vi "Set PMD wrapper.vi"(6 "pDummyPMDInfoOut":cluster{"uiPwmDuty1":u8, "uiPwmDuty2":u8}, 7 "bAckEna":i32, 8 "error in (no error)":errorcluster caption="错误输入（无错误）", 9 "pDummyPMDInfoIn":cluster{"uiPwmDuty1":u8, "uiPwmDuty2":u8}, 10 "dwCanNodeId":u32, 11 "dwDevIndex":u32) -> (0 "error out":errorcluster caption="错误输出", 1 "pDummyPMDInfoIn out":cluster{"uiPwmDuty1":u8, "uiPwmDuty2":u8}, 3 "function return":u32, 4 "pDummyPMDInfoOut out":cluster{"uiPwmDuty1":u8, "uiPwmDuty2":u8})   [LabVIEW 2016, in "UISimCanFunc_wrapper.lvlib"]
doc: "_declspec (dllexport) DWORD SetPMD_wrapper(DWORD dwDevIndex, DWORD dwCanNodeId,\n P_DUMMY_PMD_INFO_OBJ pDummyPMDInfoIn, BOOL bAckEna, P_DUMMY_PMD_INFO_OBJ pDummyPMDInfoOut);"
uses:
  <userlib>/UISimCanFunc_wrapper/UISimCanFunc_wrapper.lvlib
  <userlib>/UISimCanFunc_wrapper/UISimCanFunc_wrapper.dll
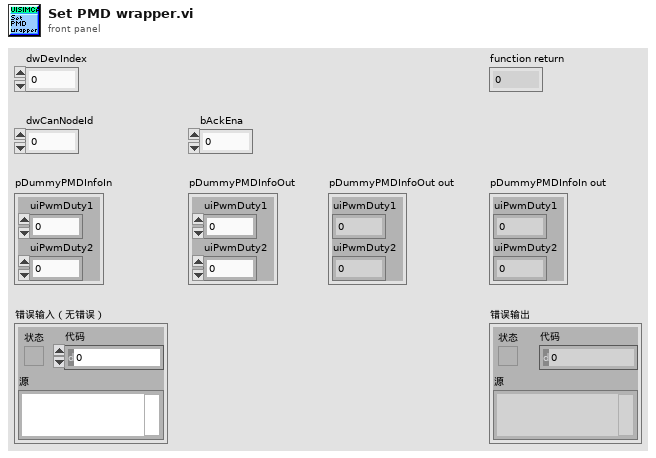
[diagram p1: front panel]
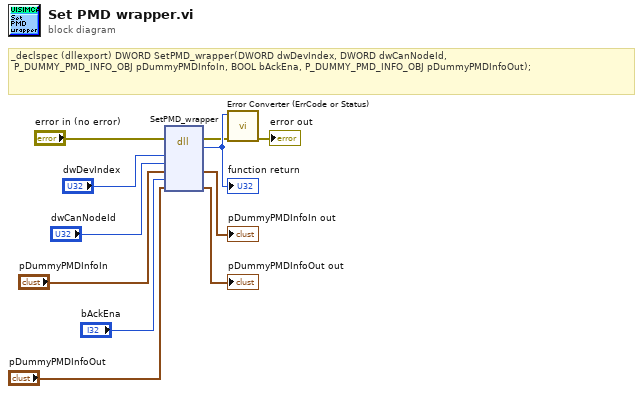
[diagram p0: block diagram]
diagram:
  # "_declspec (dllexport) DWORD SetPMD_wrapper(DWORD dwDevIndex, DWORD dwCanNodeId,\n\tP_DUMMY_PMD_INFO_OBJ pDummyPMDInfoIn, BOOL bAckEna, P_DUMMY_PMD_INFO_OBJ pDummyPMDInfoOut);"
  n1 = dll-call lib="C:/Program Files (x86)/National Instruments/LabVIEW 2016/user.lib/UISimCanFunc_wrapper/UISimCanFunc_wrapper.*" fn="SetPMD_wrapper"(error in="error in (no error)", "dwDevIndex"="dwDevIndex", "dwCanNodeId"="dwCanNodeId", "pDummyPMDInfoIn"="pDummyPMDInfoIn", "bAckEna"="bAckEna", "pDummyPMDInfoOut"="pDummyPMDInfoOut") -> (error out=w2:errorcluster, w11:u32, "pDummyPMDInfoIn"=→"pDummyPMDInfoIn out":cluster{"uiPwmDuty1":u8, "uiPwmDuty2":u8}, "pDummyPMDInfoOut"=→"pDummyPMDInfoOut out":cluster{"uiPwmDuty1":u8, "uiPwmDuty2":u8})  [unwired: 5 in, 1 out]
  "function return" <- w11
  n2 = call <userlib>:"Error Converter (ErrCode or Status).vi"("error in (no error)"=w2, "error code"=w11) -> ("error out"=→"error out":errorcluster)  [unwired: 9 in]
